vi "handler_template.vi"(8 "error in (no error)":errorcluster, 10 "Server Variables":T1 {"Energy Levels"."E1" format="%_6g"; "Phases"."ExtTriggerDelay" format="%.3g"}, 11 "HTTP Request in":T7) -> (0 "error out":errorcluster, 2 "Server Variables":T1 {"Energy Levels"."E1" format="%_6g"; "Phases"."ExtTriggerDelay" format="%.3g"}, 3 "HTTP Request out":T7)   [LabVIEW 2011]
uses:
  http_request_response.ctl
  http_request.ctl
  http_field.ctl
  http_response.ctl
  template_field.ctl
  template_field_type.ctl
  Server Variables.ctl
  Phase Parameters.ctl
  Phase Mode.ctl
  Energy Level_.ctl
  Measurement Parameters.ctl
  Results.ctl
  <vilib>/regexp/Match Regular Expression.xnode
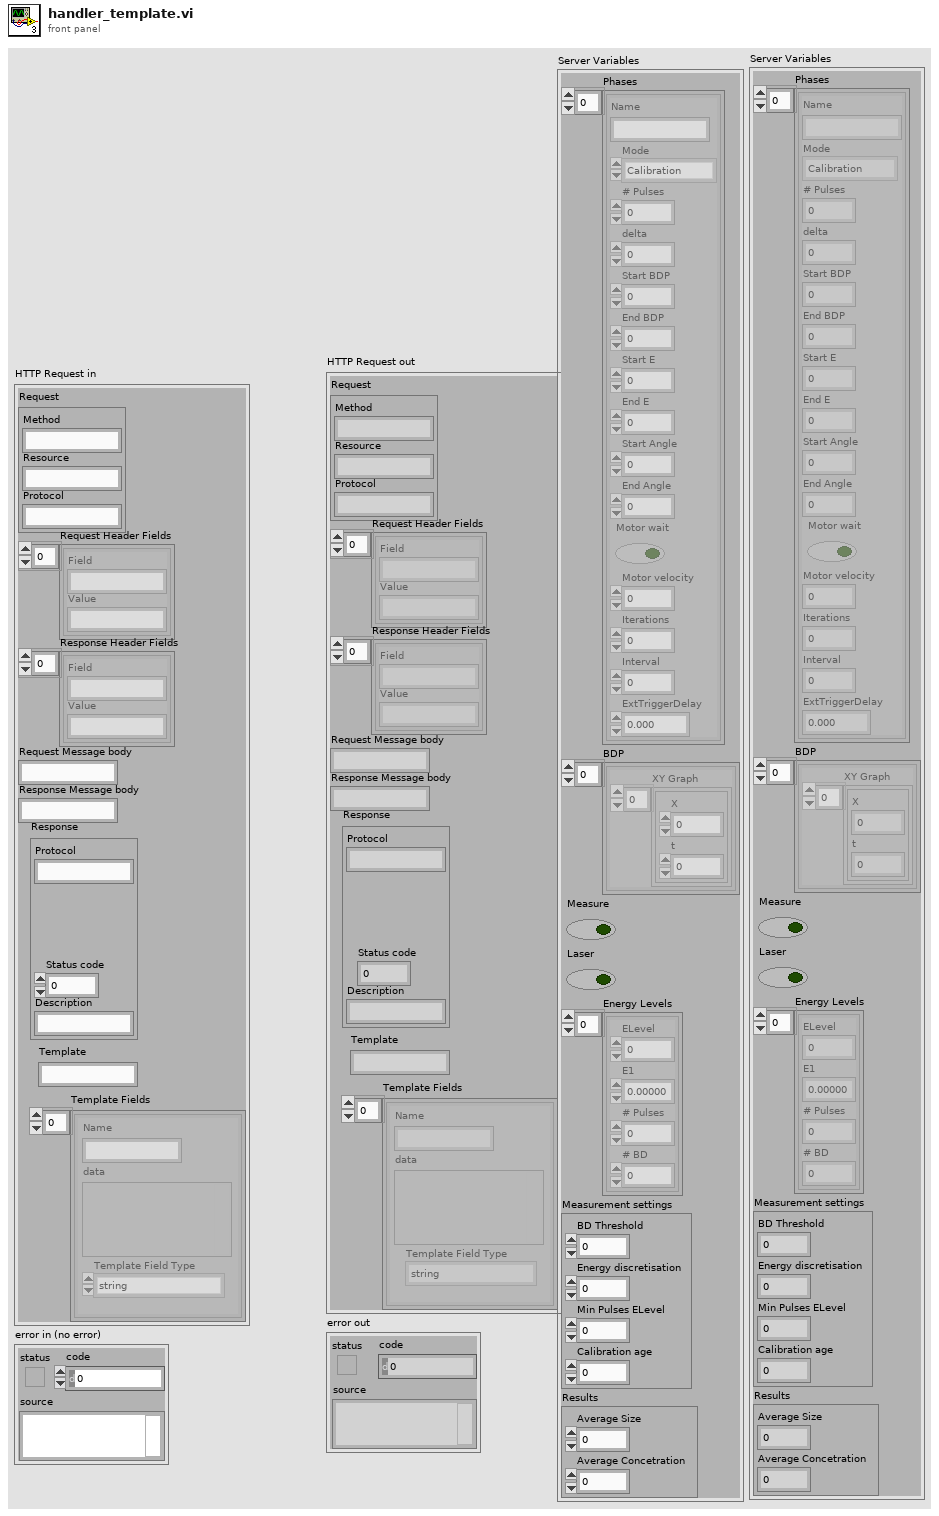
[diagram p1: front panel]
types:
  T1 = typedef "Server Variables.ctl" = cluster{"Phases":T2[], "BDP":cluster{"XY Graph":cluster{"X":dbl, "t":dbl}[]}[], "Measure":bool, "Laser":bool, "Energy Levels":T4[], "Measurement settings":T5, "Results":T6}
  T2 = typedef "Phase Parameters.ctl" = cluster{"Name":string, "Mode":T3, "# Pulses":u32, "delta":dbl, "Start BDP":dbl, "End BDP":dbl, "Start E":dbl, "End E":dbl, "Start Angle":dbl, "End Angle":dbl, "Motor wait":bool, "Motor velocity":dbl, "Iterations":dbl, "Interval":dbl, "ExtTriggerDelay":dbl}
  T3 = typedef "Phase Mode.ctl" = enum16{"Calibration", "Linear", "BDP-Fit", "Raw"}
  T4 = typedef "Energy Level_.ctl" = cluster{"ELevel":dbl, "E1":dbl, "# Pulses":i32, "# BD":i32}
  T5 = typedef "Measurement Parameters.ctl" = cluster{"BD Threshold":dbl, "Energy discretisation":i32, "Min Pulses ELevel":i32, "Calibration age":i32}
  T6 = typedef "Results.ctl" = cluster{"Average Size":dbl, "Average Concetration":dbl}
  T7 = typedef "http_request_response.ctl" = cluster{"Request":T8, "Request Header Fields":T9[], "Response Header Fields":T9[], "Request Message body":string, "Response Message body":string, "Response":T10, "Template":string, "Template Fields":T11[]}
  T8 = typedef "http_request.ctl" = cluster{"Method":string, "Resource":string, "Protocol":string}
  T9 = typedef "http_field.ctl" = cluster{"Field":string, "Value":string}
  T10 = typedef "http_response.ctl" = cluster{"Protocol":string, "Status code":dbl, "Description":string}
  T11 = typedef "template_field.ctl" = cluster{"Name":string, "Template Field Type":T12, "data":variant}
  T12 = typedef "template_field_type.ctl" = enum16{"string", "string array", "number", "number array", "cluster", "cluster array"}
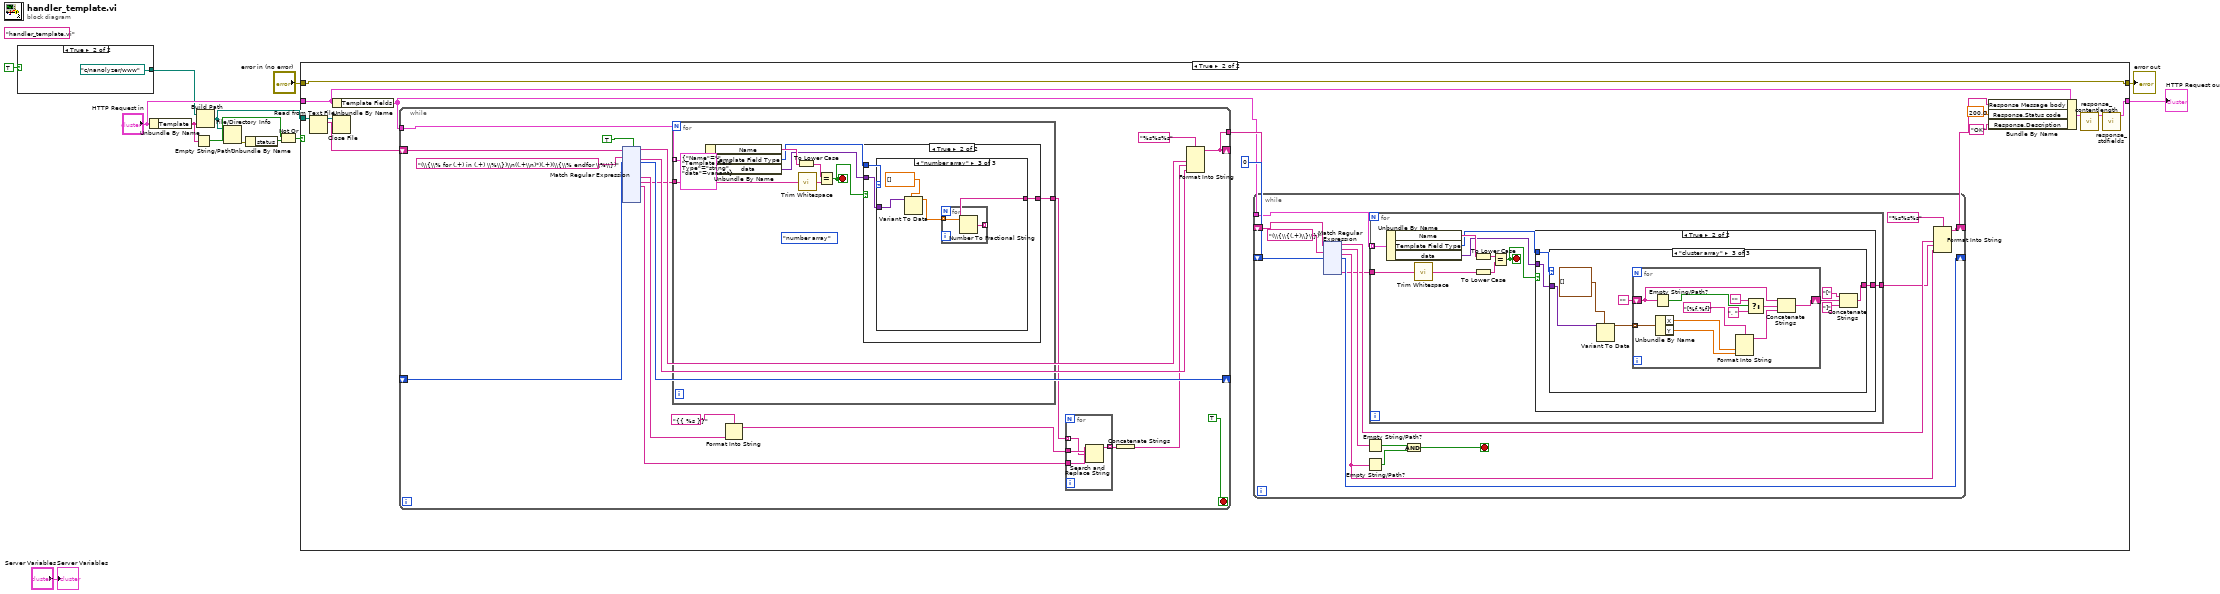
[diagram p0: block diagram]
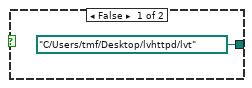
[diagram p2: hidden frame]
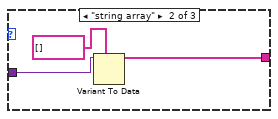
[diagram p6: hidden frame]
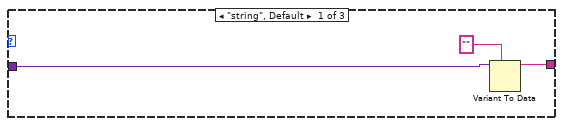
[diagram p8: hidden frame]
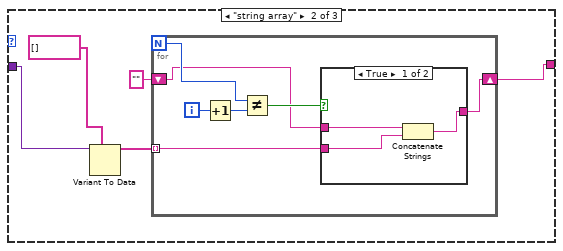
[diagram p9: hidden frame]
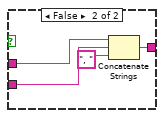
[diagram p10: hidden frame]
diagram:
  (unwired) "handler_template.vi" ("Handler name")
  n1 = case shown="True" TRUE {
    tunnel: [path "C:/Users/tmf/Desktop/lvhttpd/lvt" ("base path") path "c:/nanolyzer/www" ("base path")] -> w2
    frame False {
    }
    frame True {
    }
  }
  n2 = Unbundle By Name("HTTP Request in") -> ("Template"=w13:string)
  n3 = Empty String/Path?(string/path=w13) -> (empty?=w10:bool)
  n4 = Build Path(base path=w2, name or relative path=w13) -> (appended path=w4:path)
  n5 = File/Directory Info(path=w4) -> (error out=w12:errorcluster)  [unwired: 1 in, 6 out]
  n6 = Unbundle By Name(w12) -> ("status"=w11:bool)
  n7 = Not Or(1:w11, 2:w10) -> (0:w9:bool)
  n8 = case shown="True" w9 {
    tunnel: "HTTP Request in" -> [w16 w19]
    tunnel: [w16 w24] -> w7
    tunnel: "error in (no error)" -> [w17 w31]
    tunnel: [w17 w31] -> w5
    tunnel: w4 -> [_ w30]
    frame False {
    }
    frame True {
      n9 = Read from Text File(file (use dialog)=w30) -> (refnum out=w29:refnum<file>, text=w21:string)  [unwired: 3 in, 2 out]
      n10 = Unbundle By Name(w19) -> ("Template Fields"=w18:T11[])
      n11 = Close File(refnum=w29) -> ()  [unwired: 1 in, 2 out]
      n12 = while {
        shift-right: [w33] -> _
        shift-left: w21 -> [w49]
        shift-right: [w45] -> _
        shift-left: _ -> [w46]
        tunnel: [w33] -> w20
        tunnel: w18 -> [w32]
        stop <- TRUE stop-if-true
        n13 = xnode "Match Regular Expression"("input string"=w49, "regular expression"="(\\{\\% for (.+) in (.+) \\%\\})\\n((.+\\n)*)(.+)(\\{\\% endfor \\%\\})", "offset (0)"=w46, "multiline? (F)"=TRUE) -> ("before match"=w43:string, "after match"=w42:string, "offset past match"=w45:i32, "submatch 2"=w39:string, "submatch 3"=w37:string, "submatch 4"=w41:string)  [unwired: 2 in, 6 out]
        n14 = for {
          tunnel: w37 -> [w61]
          tunnel: [w56] -> w36
          tunnel: w32 -> [w55] mode=indexing
          stop <- w59 stop-if-true
          (unwired) T11 {"Name"="", "Template Field Type"=enum."string", "data"=variant} ("Template Field")
          (unwired) template_field_type."number array" ("Template Field Type")
          n15 = Unbundle By Name(w55) -> ("Name"=w63:string, "Template Field Type"=w58:T12, "data"=w57:variant)
          n16 = To Lower Case(string=w63) -> (all lower case string=w62:string)
          n17 = call <vilib>:"Trim Whitespace.vi"("string"=w61) -> ("trimmed string"=w60:string)  [unwired: 1 in]
          n18 = Equal?(x=w62, y=w60) -> (x = y?=w59:bool)
          n19 = case shown="True" w59 {
            tunnel: w58 -> [_ w66]
            tunnel: w57 -> [_ w65]
            tunnel: [_ w64] -> w56
            frame False {
            }
            frame True {
              n20 = case shown="\"number array\"" w66 {
                tunnel: w65 -> [_ w69 w73]
                tunnel: [_ w67 w71] -> w64
                frame "string", Default {
                }
                frame "string array" {
                  n21 = Variant To Data(type=string[] [], Variant=w69) -> (data=w67:string[])  [unwired: 1 in, 1 out]
                }
                frame "number array" {
                  n22 = Variant To Data(type=dbl[] [], Variant=w73) -> (data=w70:dbl[])  [unwired: 1 in, 1 out]
                  n23 = for {
                    tunnel: [w75] -> w71 mode=indexing
                    tunnel: w70 -> [w74] mode=indexing
                    n24 = Number To Fractional String(number=w74) -> (F-format string=w75:string)  [unwired: 3 in]
                  }
                }
              }
            }
          }
        }
        n25 = Format Into String(format string="{{ %s }}", w39) -> (resulting string=w38:string)  [unwired: 2 in, 1 out]
        n26 = for {
          tunnel: w41 -> [w54]
          tunnel: w38 -> [w53]
          tunnel: w36 -> [w52] mode=indexing
          tunnel: [w51] -> w35 mode=indexing
          n27 = Search and Replace String(input string=w54, search string=w53, replace string=w52) -> (result string=w51:string)  [unwired: 5 in, 3 out]
        }
        n28 = Concatenate Strings(w35) -> (w34:string)
        n29 = Format Into String(format string="%s%s%s", w43, w34, w42) -> (resulting string=w33:string)  [unwired: 2 in, 1 out]
      }
      n30 = while {
        shift-right: [w205] -> w28
        shift-left: w20 -> [w209]
        shift-right: [w206] -> _
        shift-left: 0 ("offset past match") -> [w207]
        tunnel: w18 -> [w195]
        stop <- w198 stop-if-true
        n31 = xnode "Match Regular Expression"("input string"=w209, "regular expression"="(\\{\\{(.+)\\}\\})", "offset (0)"=w207) -> ("before match"=w203:string, "whole match"=w197:string, "after match"=w201:string, "offset past match"=w206:i32, "submatch 2"=w196:string)  [unwired: 3 in, 2 out]
        n32 = Empty String/Path?(string/path=w197) -> (empty?=w200:bool)
        n33 = Empty String/Path?(string/path=w201) -> (empty?=w199:bool)
        n34 = for {
          tunnel: w195 -> [w219] mode=indexing
          tunnel: w196 -> [w217]
          tunnel: [w211] -> w202
          stop <- w213 stop-if-true
          n35 = Unbundle By Name(w219) -> ("Name"=w218:string, "Template Field Type"=w212:T12, "data"=w210:variant)
          n36 = call <vilib>:"Trim Whitespace.vi"("string"=w217) -> ("trimmed string"=w216:string)  [unwired: 1 in]
          n37 = To Lower Case(string=w218) -> (all lower case string=w214:string)
          n38 = To Lower Case(string=w216) -> (all lower case string=w215:string)
          n39 = Equal?(x=w214, y=w215) -> (x = y?=w213:bool)
          n40 = case shown="True" w213 {
            tunnel: w212 -> [_ w222]
            tunnel: w210 -> [_ w221]
            tunnel: [_ w220] -> w211
            frame False {
            }
            frame True {
              n41 = case shown="\"cluster array\"" w222 {
                tunnel: w221 -> [w225 w230 w252]
                tunnel: [w223 w226 w249] -> w220
                frame "string", Default {
                  n42 = Variant To Data(type="", Variant=w225) -> (data=w223:string)  [unwired: 1 in, 1 out]
                }
                frame "string array" {
                  n43 = Variant To Data(type=string[] [], Variant=w230) -> (data=w227:string[])  [unwired: 1 in, 1 out]
                  n44 = for {
                    N -> [w237]
                    tunnel: w227 -> [w233] mode=indexing
                    shift-right: [w232] -> w226
                    shift-left: "" -> [w231]
                    i -> [w236]
                    n45 = Increment(x=w236) -> (x+1=w235:i32)
                    n46 = Not Equal?(x=w237, y=w235) -> (x != y?=w234:bool)
                    n47 = case shown="True" w234 {
                      tunnel: [w239 w243] -> w232
                      tunnel: w233 -> [w240 w244]
                      tunnel: w231 -> [w238 w241]
                      frame True {
                        n48 = Concatenate Strings(w238, w240) -> (w239:string)
                      }
                      frame False {
                        n49 = Concatenate Strings(w241, w244, ", " ("string")) -> (w243:string)
                      }
                    }
                  }
                }
                frame "cluster array" {
                  n50 = Variant To Data(type=cluster{"X":dbl, "Y":dbl}[] [] ("XY Graph"), Variant=w252) -> (data=w251:cluster{"X":dbl, "Y":dbl}[])  [unwired: 1 in, 1 out]
                  n51 = for {
                    tunnel: w251 -> [w263] mode=indexing
                    shift-right: [w259] -> w248
                    shift-left: "" -> [w257]
                    n52 = Empty String/Path?(string/path=w257) -> (empty?=w256:bool)
                    n53 = Unbundle By Name(w263) -> ("X"=w261:dbl, "Y"=w260:dbl)
                    n54 = Format Into String(format string="[%f,%f]", w261, w260) -> (resulting string=w258:string)  [unwired: 2 in, 1 out]
                    n55 = Select(t="", s=w256, f=", ") -> (s? t:f=w253:string)
                    n56 = Concatenate Strings(w257, w253, w258) -> (w259:string)
                  }
                  n57 = Concatenate Strings("[" ("string"), w248, "]" ("string")) -> (w249:string)
                }
              }
            }
          }
        }
        n58 = And(x=w200, y=w199) -> (x .and. y?=w198:bool)
        n59 = Format Into String(format string="%s%s%s", w203, w202, w201) -> (resulting string=w205:string)  [unwired: 2 in, 1 out]
      }
      n60 = Bundle By Name(cluster=w19, "Response Message body"=w28, "Response.Status code"=200.0, "Response.Description"="OK") -> (w25:T7)
      n61 = call "response_contentlength.vi"("HTTP Request"=w25) -> ("HTTP Request"=w26:T7)  [unwired: 10 in]
      n62 = call "response_stdfields.vi"("HTTP Request"=w26) -> ("HTTP Request out"=w24:T7)  [unwired: 10 in]
    }
  }
  "HTTP Request out" <- w7
  "error out" <- w5
  "Server Variables" <- "Server Variables"
